vi "provideUserEvents.vi"(8 "error in (no error)":errorcluster, 11 "ViewThisComponent in":refnum<class "ViewThisComponent.lvclass">) -> (0 "error out":errorcluster, 1 "pubDataEvents":T1, 2 "stopViewUserEventCallingView":refnum<user-event>, 3 "ViewThisComponent out":refnum<class "ViewThisComponent.lvclass">)   [LabVIEW 2016, in "ViewThisComponent.lvclass"]
uses:
  ViewThisComponent.lvclass
  home/andres/ct_cmpuserevents/ComponentTemplateCore/ComponentModel/ComponentModel/View/View.lvclass
  TypedefsDataEvents/PubDataEvents.ctl
  ts_sallv_exa/DataTypes/logevent_SettingVersions.ctl
  ts_sallv_exa/DataTypes/logevent_SummaryState.ctl
  ts_sallv_exa/DataTypes/logevent_RejectedCommand.ctl
  ts_sallv_exa/DataTypes/logevent_DetailedState.ctl
  ts_sallv_exa/DataTypes/logevent_ErrorCode.ctl
  ts_sallv_exa/DataTypes/logevent_Heartbeat.ctl
  ts_sallv_exa/DataTypes/LoopTime_ms.ctl
  ts_sallv_exa/DataTypes/logevent_LoopTimeOutOfRange.ctl
  ts_sallv_exa/DataTypes/Timestamp.ctl
  ComponentTemplateCore/ComponentModel/ComponentModel/View/View.lvclass/View.ctl
  ViewThisComponent.lvclass/ViewThisComponent.ctl
  PubSubDataEvent/PubSubDataEvent.lvclass/PubSubDataEvent.ctl
  PubSubDataEvent/PubSubDataEvent.lvclass
  ComponentTemplateCore/ComponentModel/ComponentModel/View/View.lvclass
  ts_sallv_exa/SALLV_EXA.lvlib
  TypedefsDataEvents/TypedefsDataEvents.lvlib
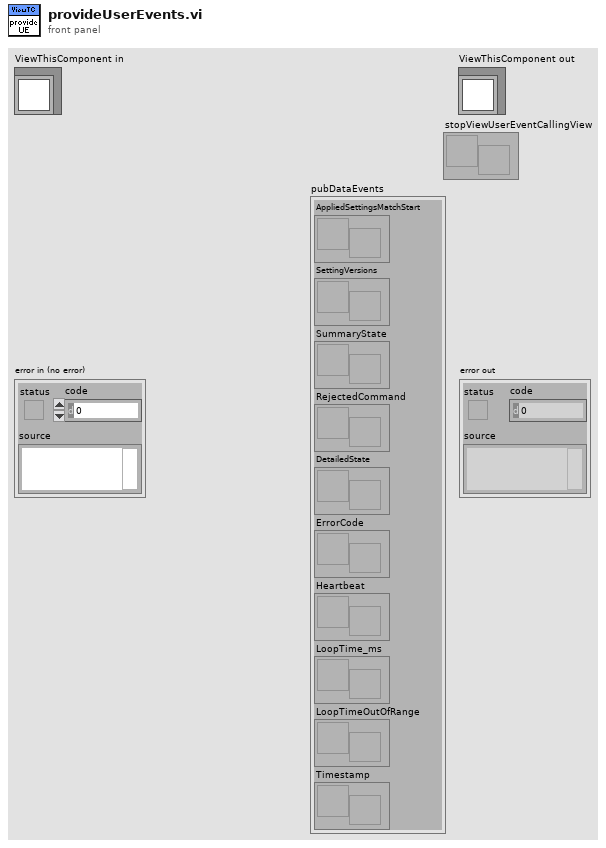
[diagram p1: front panel]
types:
  T1 = typedef "TypedefsDataEvents.lvlib/PubDataEvents.ctl" = cluster{"AppliedSettingsMatchStart":refnum<user-event>, "SettingVersions":refnum<user-event>, "SummaryState":refnum<user-event>, "RejectedCommand":refnum<user-event>, "DetailedState":refnum<user-event>, "ErrorCode":refnum<user-event>, "Heartbeat":refnum<user-event>, "LoopTime_ms":refnum<user-event>, "LoopTimeOutOfRange":refnum<user-event>, "Timestamp":refnum<user-event>}
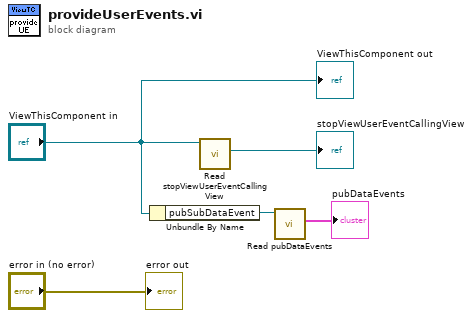
[diagram p0: block diagram]
diagram:
  n1 = Unbundle By Name("ViewThisComponent in") -> ("pubSubDataEvent"=w2:refnum<class "PubSubDataEvent.lvclass">)
  n2 = call "Read stopViewUserEventCallingView.vi"("View in"="ViewThisComponent in") -> ("stopViewUserEventCallingView"=→"stopViewUserEventCallingView":refnum<user-event>)  [unwired: 9 in, 1 out]
  n3 = call "Read pubDataEvents.vi"("PubSubDataEvent in"=w2) -> ("pubDataEvents"=→"pubDataEvents":T1)  [unwired: 9 in, 1 out]
  "error out" <- "error in (no error)"
  "ViewThisComponent out" <- "ViewThisComponent in"
